vi "readFrequency.vi"(2 "error in (no error)":errorcluster, 3 "BK1823ACounter.lvclass":refnum<class "BK1823ACounter.lvclass">) -> (0 "error out":errorcluster, 1 "BK1823ACounter.lvclass 2":refnum<class "BK1823ACounter.lvclass">)   [LabVIEW 2009, in "Hardware.lvlib" / "frequencyCounters.lvlib" / "BK1823ACounter.lvclass"]
uses:
  BK1823ACounter.lvclass
  BK1823ACounter.lvclass/BK1823ACounter.ctl
  FrequencyCounter/FrequencyCounter.lvclass
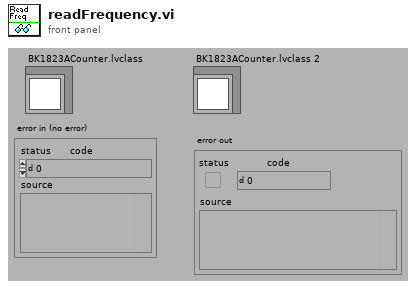
[diagram p1: front panel]
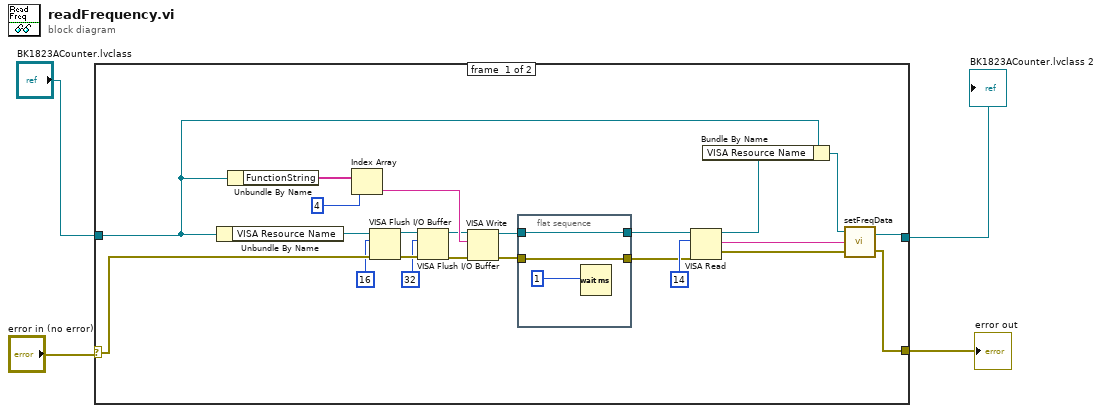
[diagram p0: block diagram]
diagram:
  n1 = case shown="No Error" "error in (no error)" {
    selector: "error in (no error)" -> [w21 w32]
    tunnel: "BK1823ACounter.lvclass" -> [w6 w31]
    tunnel: [w8 w31] -> w4
    tunnel: [w9 w32] -> w1
    frame #0 {
      n2 = Unbundle By Name(w6) -> ("VISA Resource Name"=w22:refnum<visa-resource-name>)
      n3 = Unbundle By Name(w6) -> ("FunctionString"=w27:string[])
      n4 = Index Array(array=w27, index=4) -> (element=w23:string)
      n5 = VISA Flush I/O Buffer(VISA resource name=w22, mask (16)=16, error in (no error)=w21) -> (VISA resource name out=w17:refnum<visa-resource-name>, error out=w20:errorcluster)
      n6 = VISA Flush I/O Buffer(VISA resource name=w17, mask (16)=32, error in (no error)=w20) -> (VISA resource name out=w18:refnum<visa-resource-name>, error out=w19:errorcluster)
      n7 = VISA Write(VISA resource name=w18, write buffer=w23, error in (no error)=w19) -> (VISA resource name out=w25:refnum<visa-resource-name>, error out=w24:errorcluster)  [unwired: 1 out]
      n8 = flat-sequence {
        tunnel: w25 -> [w29]
        tunnel: [w29] -> w13
        tunnel: w24 -> [w28]
        tunnel: [w28] -> w12
        frame #0 {
          n9 = Wait (ms)(milliseconds to wait=1) -> ()  [unwired: 1 out]
        }
      }
      n10 = VISA Read(VISA resource name=w13, byte count=14, error in (no error)=w12) -> (VISA resource name out=w7:refnum<visa-resource-name>, read buffer=w11:string, error out=w10:errorcluster)  [unwired: 1 out]
      n11 = Bundle By Name(cluster=w6, "VISA Resource Name"=w7) -> (w5:refnum<class "BK1823ACounter.lvclass">)
      n12 = call "setFreqData.vi"("error in (no error)"=w10, "String"=w11, "FrequencyCounter.lvclass"=w5) -> ("error out"=w9:errorcluster, "FrequencyCounter.lvclass 2"=w8:refnum<class "BK1823ACounter.lvclass">)
    }
    frame #1 {
    }
  }
  "BK1823ACounter.lvclass 2" <- w4
  "error out" <- w1
